vi "REACTOR_SHUTDOWN.vi"(8 "error in (no error)":errorcluster, 9 "Comunicaciones":T1={"Bronk mfc1"="ASRL6::INSTR", "Brk1"=FALSE, "Bronk mfc2"="ASRL6::INSTR", "Brk2"=FALSE, "Bronk mfc3"="ASRL6::INSTR", "Brk3"=FALSE, "Bronk mfc4"="ASRL6::INSTR", "Brk4"=FALSE, "Bronk mfm1"="ASRL6::INSTR", "Brkm"=FALSE, "Alicats"="ASRL6::INSTR", "Ali"=FALSE, "eVal4vias"="ASRL6::INSTR", "ev4v"=FALSE, "eVal3vias"="ASRL6::INSTR", "ev3v"=FALSE, "Cell GAS"="ASRL6::INSTR", "cgas"=FALSE, "Cell S2H"="ASRL6::INSTR", "csh2"=FALSE}) -> (0 "error out":errorcluster)   [LabVIEW 2017]
uses:
  KISSIA_COMUNICACIONES.ctl
  Z_serialTermobDisbal/Multicard III_Hardware_Module Control.ctl
  Z_modbusEurotherm P116_485/Eurotherm_Hardware_Module Control.ctl
  SERIAL ARDUINO 3VIAS VALVES/ArduinoMicro Module Control.ctl
panel:
  # "Input"
  # "Output"
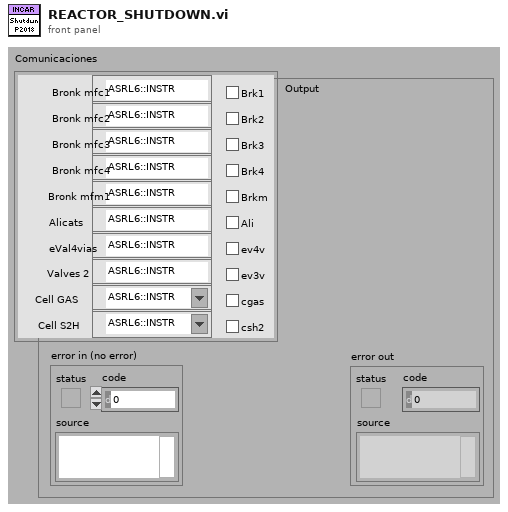
[diagram p1: front panel]
types:
  T1 = typedef "KISSIA_COMUNICACIONES.ctl" = cluster{"Bronk mfc1":refnum<visa-resource-name>, "Brk1":bool, "Bronk mfc2":refnum<visa-resource-name>, "Brk2":bool, "Bronk mfc3":refnum<visa-resource-name>, "Brk3":bool, "Bronk mfc4":refnum<visa-resource-name>, "Brk4":bool, "Bronk mfm1":refnum<visa-resource-name>, "Brkm":bool, "Alicats":refnum<visa-resource-name>, "Ali":bool, "eVal4vias":refnum<visa-resource-name>, "ev4v":bool, "eVal3vias":refnum<visa-resource-name>, "ev3v":bool, "Cell GAS":refnum<visa-resource-name>, "cgas":bool, "Cell S2H":refnum<visa-resource-name>, "csh2":bool}
  T2 = typedef "ArduinoMicro Module Control.ctl" = enum16{"Initialize", "Read Data", "Write Data", "Enable", "Disable", "Shutdown"}
  T3 = typedef "Eurotherm_Hardware_Module Control.ctl" = enum16{"Initialize", "Write SP", "Read SP+PV", "Write Rate", "Set P", "Set I", "Set D", "Shutdown"}
  T4 = typedef "Multicard III_Hardware_Module Control.ctl" = enum16{"Initialize", "Cero", "Span", "Read ugr", "Read mgr", "Read A/D", "Read T", "Number readings", "Thermocouple type", "Status", "Shutdown"}
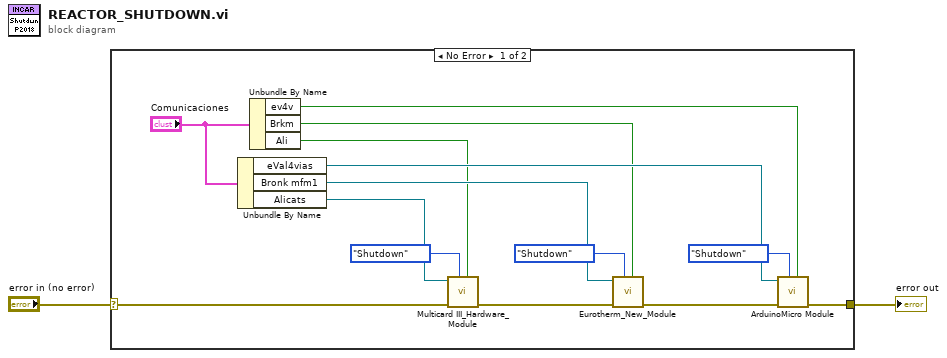
[diagram p0: block diagram]
diagram:
  n1 = case shown="No Error" "error in (no error)" {
    selector: "error in (no error)" -> [w10 w17]
    tunnel: [w8 w17] -> w1
    frame No Error {
      n2 = Unbundle By Name("Comunicaciones") -> ("eVal4vias"=w6:refnum<visa-resource-name>, "Bronk mfm1"=w11:refnum<visa-resource-name>, "Alicats"=w12:refnum<visa-resource-name>)
      n3 = Unbundle By Name("Comunicaciones") -> ("ev4v"=w3:bool, "Brkm"=w4:bool, "Ali"=w5:bool)
      n4 = call "Multicard III_Hardware_Module.vi"("Multicard (T:Enable)"=w5, "Command"=Multicard_III_Hardware_Module_Control."Shutdown", "error in (no error)"=w10, "VISA resource name"=w12) -> ("error out"=w13:errorcluster)  [unwired: 4 in, 3 out]
      n5 = call "Eurotherm_New_Module.vi"("Eurotherm (T:Enable)"=w4, "Command"=Eurotherm_Hardware_Module_Control."Shutdown", "error in (no error)"=w13, "VISA resource name"=w11) -> ("error out"=w9:errorcluster)  [unwired: 6 in, 1 out]
      n6 = call "ArduinoMicro Module.vi"("Enable"=w3, "Command"=ArduinoMicro_Module_Control."Shutdown", "error in (no error)"=w9, "VISA resource name"=w6) -> ("error out"=w8:errorcluster)  [unwired: 3 in, 4 out]
    }
    frame Error {
    }
  }
  "error out" <- w1
